vi "Control Pumps (SubVI).vi"(0 "VISA Refnum in":refnum<visa-resource-name>, 1 "Syringe Diameter (mm)":dbl, 2 "Target Vol (mL)":dbl, 5 "Address":string, 9 "Pumping Direction":bool, 11 "stop in":bool, 12 "Pumping Rate":dbl, 13 "Pumping Rate (unit)":string(combo)="MH") -> (4 "Success":bool, 6 "Pump Stopped":bool, 8 "concatenated string (Commands In)":string, 10 "read buffer":string, 14 "error out":errorcluster, 15 "return counts (Read Length)":string)   [LabVIEW 2018]
uses:
  <vilib>/Instr/_visa.llb/VISA Configure Serial Port (Instr).vi
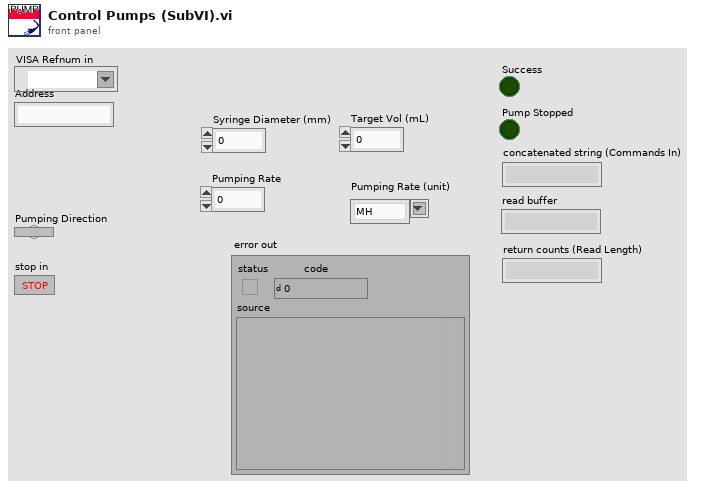
[diagram p1: front panel]
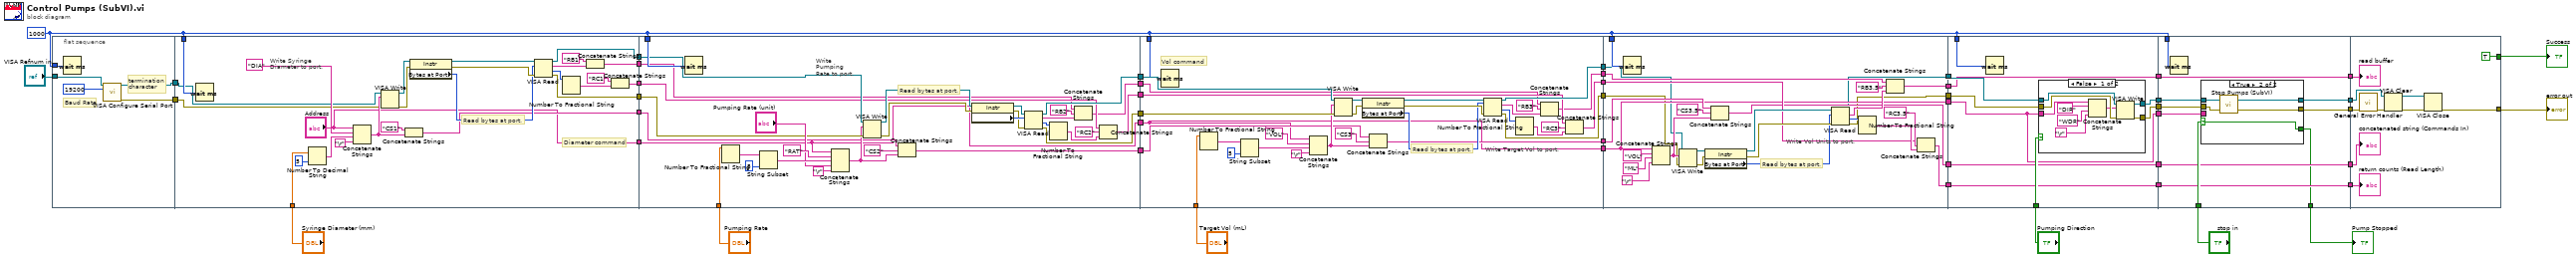
[diagram p0: block diagram]
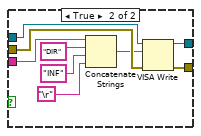
[diagram p2: hidden frame]
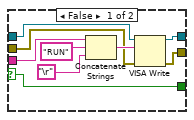
[diagram p3: hidden frame]
diagram:
  w3 = u32 1000
  n1 = flat-sequence {
    tunnel: w3 -> [w51]
    tunnel: "VISA Refnum in" -> [w50]
    tunnel: [w49] -> w2
    tunnel: [w48] -> w1
    tunnel: w3 -> [w71]
    tunnel: [w68] -> w47
    tunnel: [w67] -> w46
    tunnel: "Syringe Diameter (mm)" -> [w66]
    tunnel: [w62] -> w31
    tunnel: [w59] -> w27
    tunnel: [w56] -> w20
    tunnel: ["Address"] -> w19
    tunnel: w2 -> [w54]
    tunnel: w1 -> [w53]
    tunnel: w3 -> [w103]
    tunnel: [w102] -> w45
    tunnel: [w101] -> w44
    tunnel: w47 -> [w95]
    tunnel: w46 -> [w94]
    tunnel: "Pumping Rate" -> [w93]
    tunnel: w31 -> [w89]
    tunnel: [w88] -> w30
    tunnel: w27 -> [w85]
    tunnel: [w84] -> w26
    tunnel: [w81] -> w23
    tunnel: w20 -> [w80]
    tunnel: w19 -> [w79]
    tunnel: [w79] -> w18
    tunnel: w45 -> [w133]
    tunnel: [w130] -> w15
    tunnel: w44 -> [w132]
    tunnel: [w129] -> w13
    tunnel: w3 -> [w131]
    tunnel: "Target Vol (mL)" -> [w125]
    tunnel: w30 -> [w121]
    tunnel: [w120] -> w11
    tunnel: w26 -> [w117]
    tunnel: [w116] -> w9
    tunnel: w23 -> [w113]
    tunnel: [w112] -> w7
    tunnel: w18 -> [w111]
    tunnel: [w111] -> w5
    tunnel: w15 -> [w143]
    tunnel: [w142] -> w14
    tunnel: w13 -> [w141]
    tunnel: [w140] -> w12
    tunnel: w11 -> [w150]
    tunnel: [w149] -> w10
    tunnel: w9 -> [w148]
    tunnel: [w147] -> w8
    tunnel: w7 -> [w146]
    tunnel: [w145] -> w6
    tunnel: w5 -> [w144]
    tunnel: [w144] -> w4
    tunnel: w3 -> [w152]
    tunnel: w14 -> [w176]
    tunnel: [w174] -> w42
    tunnel: w12 -> [w175]
    tunnel: [w173] -> w43
    tunnel: "Pumping Direction" -> [w172]
    tunnel: [w171] -> w28
    tunnel: w10 -> [w171]
    tunnel: [w170] -> w24
    tunnel: w8 -> [w170]
    tunnel: [w169] -> w21
    tunnel: w6 -> [w169]
    tunnel: w4 -> [w168]
    tunnel: [w168] -> w17
    tunnel: w3 -> [w167]
    tunnel: w43 -> [w205]
    tunnel: [w204] -> w34
    tunnel: [w202] -> w33
    tunnel: w42 -> [w203]
    tunnel: [w195] -> w37
    tunnel: "stop in" -> [w201]
    tunnel: [w200] -> w29
    tunnel: w28 -> [w200]
    tunnel: [w199] -> w25
    tunnel: w24 -> [w199]
    tunnel: [w198] -> w22
    tunnel: w21 -> [w198]
    tunnel: w17 -> [w197]
    tunnel: w3 -> [w196]
    tunnel: w34 -> [w229]
    tunnel: w33 -> [w227]
    tunnel: [TRUE] -> w35
    tunnel: [w221] -> w32
    tunnel: w29 -> [w225]
    tunnel: w25 -> [w224]
    tunnel: w22 -> [w223]
    frame #0 {
      # "termination\ncharacter"
      # "Baud Rate"
      n2 = Wait (ms)(milliseconds to wait=w51) -> ()  [unwired: 1 out]
      n3 = call-poly "VISA Configure Serial Port"("VISA resource name"=w50, "baud rate (9600)"=u32 19200 ("Baud Rate (9600)")) -> ("VISA resource name out"=w49:refnum<visa-resource-name>, "error out"=w48:errorcluster)  [unwired: 12 in]
    }
    frame #1 {
      # "Diameter command"
      # "Write Syringe\nDiameter to port."
      # "Read bytes at port."
      n4 = Wait (ms)(milliseconds to wait=w71) -> ()  [unwired: 1 out]
      n5 = Number To Decimal String(number=w66, width (-)=i16 5) -> (decimal integer string=w72:string)
      n6 = Concatenate Strings("Address", "DIA", w72, "\r") -> (w57:string)
      n7 = VISA Write(VISA resource name=w54, write buffer=w57, error in (no error)=w53) -> (VISA resource name out=w78:refnum<visa-resource-name>, error out=w77:errorcluster)  [unwired: 1 out]
      n8 = Concatenate Strings("CS1", w57) -> (w56:string)
      n9 = property class="Instr"(reference=w78, error in=w77) -> (reference out=w76:refnum<visa-resource-name>, error out=w75:errorcluster, "Bytes at Port"=w74:u32)
      n10 = VISA Read(VISA resource name=w76, byte count=w74, error in (no error)=w75) -> (VISA resource name out=w67:refnum<visa-resource-name>, read buffer=w60:string, return count=w63:u32, error out=w68:errorcluster)
      n11 = Number To Fractional String(number=w63) -> (F-format string=w64:string)  [unwired: 3 in]
      n12 = Concatenate Strings("RB1", w60) -> (w59:string)
      n13 = Concatenate Strings("RC1", w64) -> (w62:string)
    }
    frame #2 {
      # "Write Pumping\nRate to port."
      # "Read bytes at port."
      n14 = Wait (ms)(milliseconds to wait=w103) -> ()  [unwired: 1 out]
      n15 = Number To Fractional String(number=w93) -> (F-format string=w97:string)  [unwired: 3 in]
      n16 = String Subset(string=w97, length (rest)=5 ("length (rest)")) -> (substring=w98:string)  [unwired: 1 in]
      n17 = Concatenate Strings(w79, "RAT", w98, "Pumping Rate (unit)", "\r") -> (w82:string)
      n18 = VISA Write(VISA resource name=w94, write buffer=w82, error in (no error)=w95) -> (VISA resource name out=w104:refnum<visa-resource-name>, error out=w105:errorcluster)  [unwired: 1 out]
      n19 = Concatenate Strings(w80, "CS2", w82) -> (w81:string)
      n20 = property class="Instr"(reference=w104, error in=w105) -> (reference out=w106:refnum<visa-resource-name>, error out=w107:errorcluster, "Serial Settings:Number of Bytes at Serial Port"=w108:u32)
      n21 = VISA Read(VISA resource name=w106, byte count=w108, error in (no error)=w107) -> (VISA resource name out=w101:refnum<visa-resource-name>, read buffer=w86:string, return count=w90:u32, error out=w102:errorcluster)
      n22 = Number To Fractional String(number=w90) -> (F-format string=w91:string)  [unwired: 3 in]
      n23 = Concatenate Strings(w85, "RB2", w86) -> (w84:string)
      n24 = Concatenate Strings(w89, "RC2", w91) -> (w88:string)
    }
    frame #3 {
      # "Vol command"
      # "Write Target Vol to port."
      # "Read bytes at port."
      n25 = Wait (ms)(milliseconds to wait=w131) -> ()  [unwired: 1 out]
      n26 = Number To Fractional String(number=w125) -> (F-format string=w127:string)  [unwired: 3 in]
      n27 = String Subset(string=w127, length (rest)=i16 5 ("width (-)")) -> (substring=w128:string)  [unwired: 1 in]
      n28 = Concatenate Strings(w111, "VOL", w128, "\r") -> (w114:string)
      n29 = VISA Write(VISA resource name=w132, write buffer=w114, error in (no error)=w133) -> (VISA resource name out=w139:refnum<visa-resource-name>, error out=w138:errorcluster)  [unwired: 1 out]
      n30 = property class="Instr"(reference=w139, error in=w138) -> (reference out=w137:refnum<visa-resource-name>, error out=w136:errorcluster, "Bytes at Port"=w135:u32)
      n31 = Concatenate Strings(w113, "CS3", w114) -> (w112:string)
      n32 = VISA Read(VISA resource name=w137, byte count=w135, error in (no error)=w136) -> (VISA resource name out=w129:refnum<visa-resource-name>, read buffer=w118:string, return count=w122:u32, error out=w130:errorcluster)
      n33 = Number To Fractional String(number=w122) -> (F-format string=w123:string)  [unwired: 3 in]
      n34 = Concatenate Strings(w117, "RB3", w118) -> (w116:string)
      n35 = Concatenate Strings(w121, "RC3", w123) -> (w120:string)
    }
    frame #4 {
      # "Write Vol Units to port."
      # "Read bytes at port."
      n36 = Wait (ms)(milliseconds to wait=w152) -> ()  [unwired: 1 out]
      n37 = Concatenate Strings(w144, "VOL", "ML", "\r") -> (w154:string)
      n38 = VISA Write(VISA resource name=w141, write buffer=w154, error in (no error)=w143) -> (VISA resource name out=w166:refnum<visa-resource-name>, error out=w165:errorcluster)  [unwired: 1 out]
      n39 = property class="Instr"(reference=w166, error in=w165) -> (reference out=w164:refnum<visa-resource-name>, error out=w163:errorcluster, "Bytes at Port"=w162:u32)
      n40 = Concatenate Strings(w146, "CS3.5", w154) -> (w145:string)
      n41 = VISA Read(VISA resource name=w164, byte count=w162, error in (no error)=w163) -> (VISA resource name out=w140:refnum<visa-resource-name>, read buffer=w156:string, return count=w158:u32, error out=w142:errorcluster)
      n42 = Number To Fractional String(number=w158) -> (F-format string=w159:string)  [unwired: 3 in]
      n43 = Concatenate Strings(w148, "RB3.5", w156) -> (w147:string)
      n44 = Concatenate Strings(w150, "RC3.5", w159) -> (w149:string)
    }
    frame #5 {
      n45 = Wait (ms)(milliseconds to wait=w167) -> ()  [unwired: 1 out]
      n46 = case shown="False" w172 {
        tunnel: w176 -> [w185 w194]
        tunnel: w175 -> [w184 w193]
        tunnel: [w183 w192] -> w174
        tunnel: [w182 w191] -> w173
        tunnel: w168 -> [w177 w186]
        frame False {
          n47 = Concatenate Strings(w177, "DIR", "WDR", "\r") -> (w178:string)
          n48 = VISA Write(VISA resource name=w184, write buffer=w178, error in (no error)=w185) -> (VISA resource name out=w182:refnum<visa-resource-name>, error out=w183:errorcluster)  [unwired: 1 out]
        }
        frame True {
          n49 = Concatenate Strings(w186, "DIR", "INF", "\r") -> (w190:string)
          n50 = VISA Write(VISA resource name=w193, write buffer=w190, error in (no error)=w194) -> (VISA resource name out=w191:refnum<visa-resource-name>, error out=w192:errorcluster)  [unwired: 1 out]
        }
      }
    }
    frame #6 {
      n51 = Wait (ms)(milliseconds to wait=w196) -> ()  [unwired: 1 out]
      n52 = case shown="True" w201 {
        selector: w201 -> [w206 w215]
        tunnel: w203 -> [w211 w219]
        tunnel: w205 -> [w210 w218]
        tunnel: [w209 w217] -> w204
        tunnel: [w208 w216] -> w202
        tunnel: w197 -> [w207 _]
        tunnel: [w206 w215] -> w195
        frame False {
          n53 = Concatenate Strings(w207, "RUN", "\r") -> (w212:string)
          n54 = VISA Write(VISA resource name=w210, write buffer=w212, error in (no error)=w211) -> (VISA resource name out=w209:refnum<visa-resource-name>, error out=w208:errorcluster)  [unwired: 1 out]
        }
        frame True {
          n55 = call "Stop Pumps (SubVI).vi"("error out 2"=w219, "VISA resource name out 2"=w218) -> ("error out"=w216:errorcluster, "VISA resource name out"=w217:refnum<visa-resource-name>)
        }
      }
    }
    frame #7 {
      n56 = call <vilib>:"General Error Handler.vi"("error in (no error)"=w227) -> ("error out"=w226:errorcluster)  [unwired: 2 in, 12 out]
      n57 = VISA Clear(VISA resource name=w229, error in (no error)=w226) -> (VISA resource name out=w222:refnum<visa-resource-name>, error out=w220:errorcluster)
      n58 = VISA Close(VISA resource name=w222, error in (no error)=w220) -> (error out=w221:errorcluster)
      "return counts (Read Length)" <- w225
      "read buffer" <- w224
      "concatenated string (Commands In)" <- w223
    }
  }
  "Pump Stopped" <- w37
  "Success" <- w35
  "error out" <- w32
